vi "Entrain2.vi"() -> ()   [LabVIEW 2013]
uses:
  Data.ctl
  <vilib>/Platform/TimedLoop/XDataNode/timing_clust.ctl
  <vilib>/Platform/TimedLoop/XDataNode/nitl_modes.ctl
  <vilib>/Platform/TimedLoop/XDataNode/wakeup.ctl
  <vilib>/DAQmx/read.llb/DAQmx Read (Analog 1D Wfm NChan NSamp).vi
  <vilib>/DAQmx/miscellaneous.llb/DAQmx Fill In Error Info.vi
  <vilib>/Platform/TimedLoop/XDataNode/XDataNode.xnode
  <vilib>/Platform/TimedLoop/XDataNode/XDNodeRunTimeDep.lvlib
panel:
  in  "clear":bool
  out "Phase graph":cluster{"Y":dbl[], dbl[]}[](graph)
  in  "Which phase":enum16{"Sine", "Stimulus"}(ring)
  out "noiseamp":dbl[unit] caption="Noise amplitude"
  out "sinamp":dbl[unit] caption="Sine amplitude"
  out "sinfreq":dbl[unit] caption="Sine frequency"
  out "Data":waveform(dbl)[](graph)
  in  "stop":bool
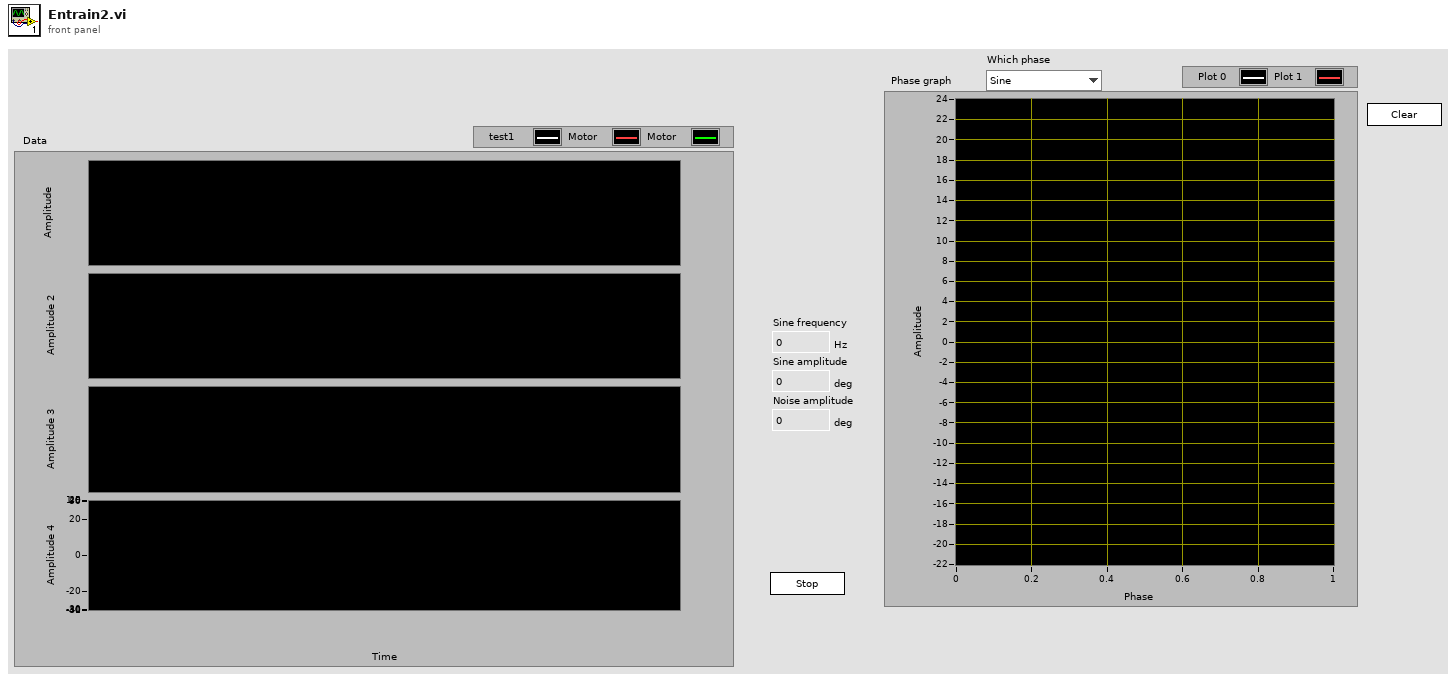
[diagram p1: front panel]
types:
  T1 = typedef "Data.ctl" = cluster{"voltage":waveform(dbl)[]}
  T2 = typedef "Sampling info.ctl" = cluster{"Channels":T3[], "Sampling freq":dbl, "Output freq":dbl, "Update freq":dbl, "Steps per rev":i32, "Counts per rev":i32, "Amplifier":string, "Motor driver":string, "Step bit":u8, "Max speed":dbl, "Max accel":dbl, "Pos gain":dbl, "Vel gain":dbl, "counter":tag}
  T3 = typedef "Channel.ctl" = cluster{"Name":string, "Chan":tag, "Gain":u16, "Lo cutoff":dbl, "Hi cutoff":dbl, "Notch":bool}
  T4 = typedef "Stim phases.ctl" = cluster{"sinephase":waveform(dbl), "sinecycles":waveform(dbl), "stimphase":waveform(dbl), "stimcycles":waveform(dbl)}
  T5 = typedef "Stimulus.ctl" = cluster{"type":T6, "sinfreq start":dbl, "sinfreq end":dbl, "sinamp start":dbl, "sinamp end":dbl, "noise freq lo":dbl, "noise freq hi":dbl, "noiseamp start":dbl, "noiseamp end":dbl, "stimdur":dbl, "before dur":dbl, "after dur":dbl, "pulse data":T7}
  T6 = typedef "Stimulus type.ctl" = enum16{"Zero", "Sine", "Frequency sweep", "Two frequency", "Amplitude sweep", "Pulses", "Shifts"}
  T7 = typedef "Pulse data.ctl" = cluster{"time":dbl[], "phase":dbl[], "dir/phase2":dbl[], "amplitude":dbl[], "duration":dbl[]}
  T8 = typedef "File refs.ctl" = cluster{"file":T9, "voltage data":i32, "motor data":i32, "command data":i32, "encoder data":i32}
  T9 = typedef "hid_t.ctl" = i32
  T10 = typedef "XDNodeRunTimeDep.lvlib/timing_clust.ctl" = cluster{"Expected End [f-1]":u64, "Actual End [f-1]":u64, "Finished Late? [f-1]":bool, "Expected End [i-1]":u64, "Actual End [i-1]":u64, "Finished Late? [i-1]":bool, "Expected Start [i]":u64, "Actual Start [i]":u64, "Expected Start [f]":u64, "Actual Start [f]":u64, "Source Name":string, "Structure Name":string, "Period":i64, "Deadline":i64, "Offset":i64, "Start":i64, "Priority":i32, "Timeout":i32, "Mode":T11, "Wakeup Reason":T12, "Error":errorcluster, "Source Type":string, "Secondary Source Type":string, "Global End Time":u64, "Global Start Time":u64, "Frame Duration":u64, "Iteration Duration":u64, "Assigned CPU":i32, "I/O Scan Engine Mode":u32}
  T11 = typedef "XDNodeRunTimeDep.lvlib/nitl_modes.ctl" = enum32{"No Change", "Process missed periods, maintain original phase", "Discard missed periods, maintain original phase", "Process missed periods, ignore original phase", "Discard missed periods, ignore original phase"}
  T12 = typedef "XDNodeRunTimeDep.lvlib/wakeup.ctl" = enum32{"Normal", "Aborted", "Asynchronous wakeup", "Timing source error", "Timed loop error", "Timeout"}
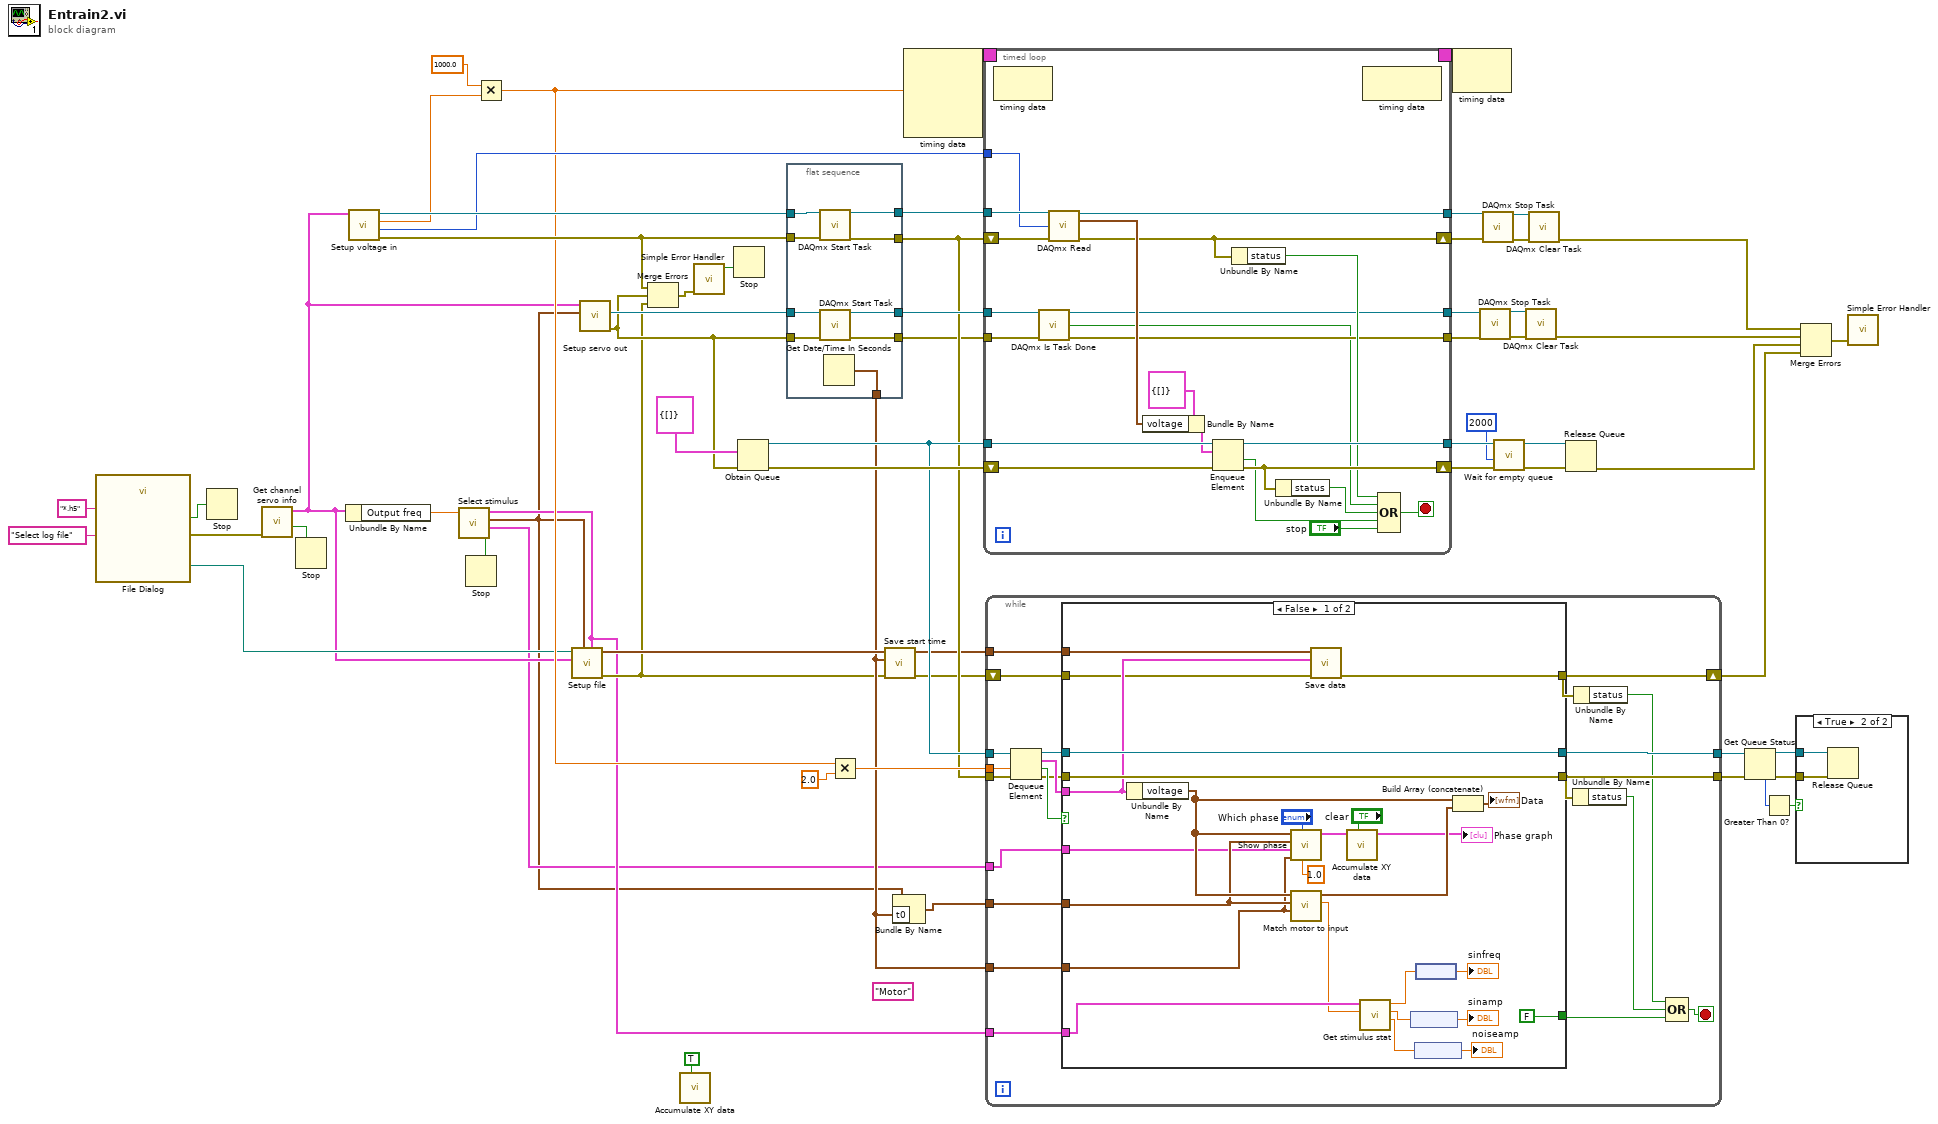
[diagram p0: block diagram]
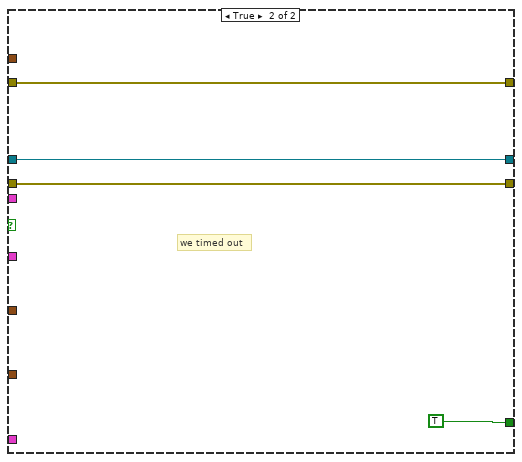
[diagram p3: hidden frame]
diagram:
  (unwired) "Motor" ("name")
  n1 = call "File Dialog"("prompt"="Select log file", "pattern (all files)"="*.h5") -> ("selected path"=w20:path, "cancelled"=w61:bool, "error out"=w60:errorcluster)  [unwired: 10 in, 1 out]
  n2 = Stop(stop? (T)=w61) -> ()
  n3 = call "Get channel servo info.vi"("error in"=w60) -> ("Cancelled"=w64:bool, "Sampling info"=w19:T2)  [unwired: 8 in, 1 out]
  n4 = Stop(stop? (T)=w64) -> ()
  n5 = Unbundle By Name(w19) -> ("Output freq"=w21:dbl)
  n6 = call "Setup voltage in.vi"("Sampling info in"=w19) -> ("error out"=w54:errorcluster, "number of input samples"=w48:i32, "update period"=w50:dbl, "task out"=w57:refnum<k21>)  [unwired: 6 in]
  n7 = call "Select stimulus.vi"("Output freq (Hz)"=w21) -> ("cancelled"=w5:bool, "stimphases"=w4:T4, "output waveform"=w3:waveform(dbl), "Stimulus"=w6:T5)  [unwired: 6 in]
  n8 = Stop(stop? (T)=w5) -> ()
  n9 = Multiply(x=1000.0, y=w50) -> (x*y=w37:dbl)
  n10 = call "Setup file.vi"("Stimulus"=w6, "motor"=w3, "Sampling data"=w19, "selected path"=w20) -> ("error out"=w9:errorcluster, "file refs"=w11:T8)  [unwired: 4 in, 2 out]
  n11 = call "Setup servo out.vi"("signal"=w3, "Sampling info in"=w19) -> ("error out"=w25:errorcluster, "task out"=w56:refnum<k21>)  [unwired: 7 in, 1 out]
  n12 = Merge Errors(w54, w25, w9) -> (w53:errorcluster)
  n13 = call "Accumulate XY data.vi"("reset"=TRUE) -> ()  [unwired: 10 in, 1 out]
  n14 = call <vilib>:"Simple Error Handler.vi"("error in (no error)"=w53) -> ("error?"=w52:bool)  [unwired: 4 in, 4 out]
  n15 = Stop(stop? (T)=w52) -> ()
  n16 = Obtain Queue(element data type=T1 {"voltage"=[]} ("data"), error in (no error)=w25) -> (queue out=w45:refnum<queue>, error out=w46:errorcluster)  [unwired: 3 in, 1 out]
  n17 = flat-sequence {
    tunnel: w57 -> [w73]
    tunnel: w56 -> [w72]
    tunnel: [w71] -> w10
    tunnel: [w70] -> w55
    tunnel: w54 -> [w69]
    tunnel: w25 -> [w68]
    tunnel: [w67] -> w51
    tunnel: [w66] -> w24
    tunnel: [w65] -> w23
    frame #0 {
      n18 = call <vilib>:"DAQmx Start Task.vi"("task/channels in"=w73, "error in"=w69) -> ("task out"=w70:refnum<k21>, "error out"=w66:errorcluster)  [unwired: 12 in]
      n19 = call <vilib>:"DAQmx Start Task.vi"("task/channels in"=w72, "error in"=w68) -> ("task out"=w67:refnum<k21>, "error out"=w65:errorcluster)  [unwired: 12 in]
      n20 = Get Date/Time In Seconds() -> (seconds since 1Jan1904=w71:timestamp)
    }
  }
  n21 = Multiply(x=w37, y=2.0) -> (x*y=w32:dbl)
  n22 = call "Save start time.vi"("error in (no error)"=w9, "Start time"=w10, "file refs"=w11) -> ("error out"=w7:errorcluster, "file refs out"=w8:T8)  [unwired: 7 in]
  n23 = Bundle By Name(cluster=w3, "t0"=w10) -> (w2:waveform(dbl))
  n24 = node-c288(w37) -> (w59:T10)  [unwired: 3 in]
  n25 = timed-loop {
    timing: w59 -> [_]
    timing-out: [_] -> w58
    tunnel: w55 -> [w95]
    tunnel: w51 -> [w78]
    tunnel: w48 -> [w94]
    tunnel: w45 -> [w92]
    tunnel: [w89] -> w44
    tunnel: [w86] -> w30
    tunnel: [w76] -> w38
    shift-right: [w84] -> w29
    shift-left: w46 -> [w88]
    shift-right: [w85] -> w43
    shift-left: w24 -> [w93]
    tunnel: w23 -> [w77]
    tunnel: [w75] -> w22
    stop <- w79 stop-if-true
    n26 = node-c288() -> ()  [unwired: 1 in, 1 out]
    n27 = call <vilib>:"DAQmx Is Task Done.vi"("task/channels in"=w78, "error in"=w77) -> ("task out"=w76:refnum<k21>, "task done?"=w74:bool, "error out"=w75:errorcluster)  [unwired: 11 in]
    n28 = call-poly <vilib>:"DAQmx Read.vi"("task/channels in"=w95, "number of samples per channel"=w94, "error in"=w93) -> ("task out"=w89:refnum<k21>, "data"=w90:waveform(dbl)[], "error out"=w85:errorcluster)  [unwired: 10 in]
    n29 = Bundle By Name(cluster=T1 {"voltage"=[]} ("data"), "voltage"=w90) -> (w87:T1)
    n30 = Enqueue Element(queue=w92, element=w87, error in (no error)=w88) -> (queue out=w86:refnum<queue>, timed out?=w81:bool, error out=w84:errorcluster)  [unwired: 1 in]
    n31 = Unbundle By Name(w85) -> ("status"=w83:bool)
    n32 = Unbundle By Name(w84) -> ("status"=w82:bool)
    n33 = node-c288() -> ()  [unwired: 1 in, 1 out]
    n34 = Compound Arithmetic op=OR(w83, w74, w82, w81, "stop") -> (w79:bool)
  }
  n35 = while {
    tunnel: w45 -> [w117]
    tunnel: w32 -> [w116]
    tunnel: [w113] -> w17
    tunnel: [w109] -> w16
    tunnel: w24 -> [w110]
    tunnel: w2 -> [w105]
    tunnel: w10 -> [w104]
    tunnel: w8 -> [w103]
    shift-right: [w101] -> w18
    shift-left: w7 -> [w102]
    tunnel: w6 -> [w99]
    tunnel: w4 -> [w98]
    stop <- w108 stop-if-true
    n36 = Dequeue Element(queue=w117, timeout in ms (-1)=w116, error in (no error)=w110) -> (queue out=w112:refnum<queue>, element=w115:T1, timed out?=w114:bool, error out=w111:errorcluster)
    n37 = case shown="False" w114 {
      tunnel: w115 -> [w137 _]
      tunnel: [FALSE TRUE] -> w107
      tunnel: [w142 w146] -> w113
      tunnel: w112 -> [w142 w146]
      tunnel: [w141 w145] -> w109
      tunnel: w111 -> [w141 w145]
      tunnel: w105 -> [w125 _]
      tunnel: w104 -> [w123 _]
      tunnel: w103 -> [w138 _]
      tunnel: w102 -> [w136 w144]
      tunnel: [w135 w144] -> w101
      tunnel: w99 -> [w134 _]
      tunnel: w98 -> [w124 _]
      frame False {
        n38 = Unbundle By Name(w137) -> ("voltage"=w126:waveform(dbl)[])
        n39 = call "Show phase.vi"("offset"=1.0, "Which phase"="Which phase", "start time"=w123, "stimphases"=w124, "motor"=w125, "voltage"=w126) -> ("plots"=w121:cluster{"Y":dbl[], dbl[]}[])  [unwired: 5 in]
        n40 = call "Match motor to input.vi"("start time"=w123, "motor"=w125, "voltage"=w126) -> ("time"=w133:dbl, "motor subset"=w140:waveform(dbl))  [unwired: 7 in]
        n41 = call "Save data.vi"("error in (no error)"=w136, "data"=w137, "file refs"=w138) -> ("error out"=w135:errorcluster)  [unwired: 8 in]
        n42 = call "Accumulate XY data.vi"("reset"="clear", "plots"=w121) -> ("plots out"=→"Phase graph":cluster{dbl[], dbl[]}[])  [unwired: 9 in]
        n43 = call "Get stimulus stat.vi"("time"=w133, "Stimulus"=w134) -> ("noiseamp"=w127:dbl, "sinamp"=w128:dbl, "sinfreq"=w132:dbl)  [unwired: 7 in]
        n44 = node(w128) -> (→"sinamp":dbl[unit])
        n45 = node(w127) -> (→"noiseamp":dbl[unit])
        n46 = node(w132) -> (→"sinfreq":dbl[unit])
        n47 = Build Array (concatenate)(w126, w140) -> (→"Data":waveform(dbl)[])
      }
      frame True {
        # "we timed out"
      }
    }
    n48 = Unbundle By Name(w109) -> ("status"=w106:bool)
    n49 = Unbundle By Name(w101) -> ("status"=w100:bool)
    n50 = Compound Arithmetic op=OR(w100, w106, w107) -> (w108:bool)
  }
  n51 = node-c288(w58) -> ()  [unwired: 1 out]
  n52 = call <vilib>:"DAQmx Stop Task.vi"("task/channels in"=w38, "error in"=w22) -> ("task out"=w39:refnum<k21>, "error out"=w40:errorcluster)  [unwired: 12 in]
  n53 = call <vilib>:"DAQmx Stop Task.vi"("task/channels in"=w44, "error in"=w43) -> ("task out"=w42:refnum<k21>, "error out"=w41:errorcluster)  [unwired: 12 in]
  n54 = call "Wait for empty queue.vi"("error in (no error)"=w29, "timeout"=2000, "Queue in"=w30) -> ("error out"=w26:errorcluster, "Queue out"=w27:refnum<queue>)  [unwired: 7 in]
  n55 = call <vilib>:"DAQmx Clear Task.vi"("task in"=w39, "error in"=w40) -> ("error out"=w35:errorcluster)  [unwired: 13 in]
  n56 = call <vilib>:"DAQmx Clear Task.vi"("task in"=w42, "error in"=w41) -> ("error out"=w36:errorcluster)  [unwired: 13 in]
  n57 = Release Queue(queue=w27, error in (no error)=w26) -> (error out=w34:errorcluster)  [unwired: 1 in, 2 out]
  n58 = Get Queue Status(queue=w17, error in (no error)=w16) -> (queue out=w12:refnum<queue>, error out=w13:errorcluster, # elements in queue=w14:i32)  [unwired: 1 in, 5 out]
  n59 = Greater Than 0?(x=w14) -> (x > 0?=w15:bool)
  n60 = case shown="True" w15 {
    tunnel: w13 -> [_ w149]
    tunnel: w12 -> [_ w148]
    frame False {
    }
    frame True {
      n61 = Release Queue(queue=w148, error in (no error)=w149) -> ()  [unwired: 1 in, 3 out]
    }
  }
  n62 = Merge Errors(w36, w35, w34, w18) -> (w33:errorcluster)
  n63 = call <vilib>:"Simple Error Handler.vi"("error in (no error)"=w33) -> ()  [unwired: 4 in, 5 out]
